vi "Initialize Session.vi"   [LabVIEW 2020, in "SLSC.lvlib"]
doc: "Initializes an SLSC session."
uses:
  <vilib>/SLSC/SLSC.lvlib
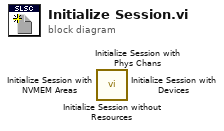
[diagram p0: block diagram]
diagram:
  n1 = call <vilib>:"Initialize Session without Resources.vi"() -> ()  [unwired: 14 in, 2 out]
  n2 = call <vilib>:"Initialize Session with Phys Chans.vi"() -> ()  [unwired: 14 in, 2 out]
  n3 = call <vilib>:"Initialize Session with NVMEM Areas.vi"() -> ()  [unwired: 14 in, 2 out]
  n4 = call <vilib>:"Initialize Session with Devices.vi"() -> ()  [unwired: 14 in, 2 out]
